vi "ParseSWI.vi"(8 "error in (no error)":errorcluster, 9 "Master Device in":refnum<class "Master Device.lvclass">, 10 "Current Variables":T1[](array[typedef]), 11 "SRS_SG380 in":refnum<class "SRS_SG380.lvclass">) -> (0 "error out":errorcluster, 2 "Master Device out":refnum<class "Master Device.lvclass">, 3 "SRS_SG380 out":refnum<class "SRS_SG380.lvclass">)   [LabVIEW 2013, in "SRS_SG380.lvclass"]
doc: "All specific devices will override ParseSWI method (i.e. you can delete the parent call)\n (1) Get devices data from private data\n (2) Get Slave Info (Ramp List) from Master Device\n (3) Parse data into \"prepared HWI\" which is in reverse order to match Ramp List."
uses:
  SRS_SG380.lvclass
  TypeDefs/Active procedure variables.ctl
  Master Device/Master Device.lvclass
  SRS_SG380.lvclass/SRS_SG380.ctl
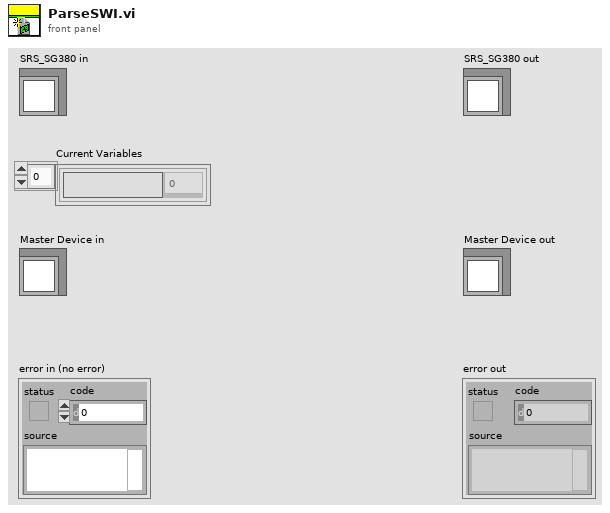
[diagram p1: front panel]
types:
  T1 = typedef "Active procedure variables.ctl" = cluster{"Procedure variable":string, "Value":dbl}
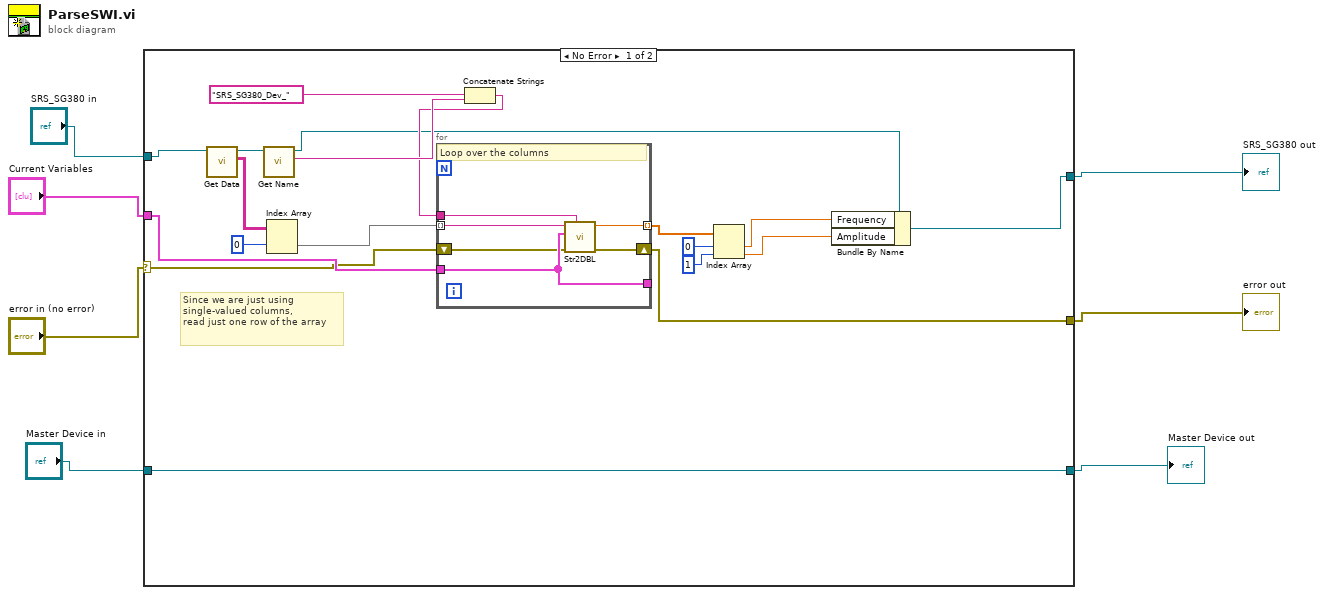
[diagram p0: block diagram]
diagram:
  n1 = case shown="No Error" "error in (no error)" {
    selector: "error in (no error)" -> [w11 w35]
    tunnel: [w10 w35] -> w1
    tunnel: "Master Device in" -> [w26 w34]
    tunnel: [w26 w34] -> w3
    tunnel: "SRS_SG380 in" -> [w25 w33]
    tunnel: [w8 w33] -> w2
    tunnel: "Current Variables" -> [w20 _]
    frame No Error {
      # "Since we are just using single-valued columns, \nread just one row of the array"
      n2 = call-dynamic "Get Data.vi"("Device in"=w25) -> ("Table Indicator"=w19:string[][], "Device out"=w24:refnum<class "SRS_SG380.lvclass">)  [unwired: 7 in, 1 out]
      n3 = call-dynamic "Get Name.vi"("Device in"=w24) -> ("Name"=w23:string, "Device out"=w9:refnum<class "SRS_SG380.lvclass">)  [unwired: 8 in, 1 out]
      n4 = Index Array(array=w19, index (row)=0) -> (element=w12:string[])  [unwired: 1 in]
      n5 = Concatenate Strings("SRS_SG380_Dev_", w23) -> (w21:string)
      n6 = for {
        tunnel: w21 -> [w28]
        tunnel: w20 -> [w29]
        tunnel: w12 -> [w32] mode=indexing
        tunnel: [w31] -> w17 mode=indexing
        shift-right: [w30] -> w10
        shift-left: w11 -> [w27]
        tunnel: [w29] -> _
        # "Loop over the columns"
        n7 = call "Str2DBL.vi"("Error Locator"=w28, "error in (no error)"=w27, "Current Variable settings"=w29, "formula"=w32) -> ("error out"=w30:errorcluster, "y value"=w31:dbl)  [unwired: 4 in]
      }
      n8 = Index Array(array=w17, index #1=0 ("index"), index #2=1 ("index")) -> (element #1=w14:dbl, element #2=w13:dbl)
      n9 = Bundle By Name(cluster=w9, "Frequency"=w14, "Amplitude"=w13) -> (w8:refnum<class "SRS_SG380.lvclass">)
    }
    frame Error {
    }
  }
  "error out" <- w1
  "SRS_SG380 out" <- w2
  "Master Device out" <- w3
